vi "S2C_PCIe7841_Proc_AnalogWrite.vi"(8 "Error In":errorcluster, 11 "Data":string) -> (0 "Error Out":errorcluster)   [LabVIEW 2015]
uses:
  S2C_PCIe7841_Proc_Globals.vi
  <vilib>/Utility/error.llb/Error Cluster From Error Code.vi
  <vilib>/rvi/errors/niLvFpgaAdjustHostInterfaceError.vi
  <vilib>/rvi/interface/nirviReadWriteControl/nirviReadWriteControl.xnode
  <vilib>/rvi/interface/Simulation/niFpgaSimulationCallBeginRW.vi
  NiFpgaLv.dll
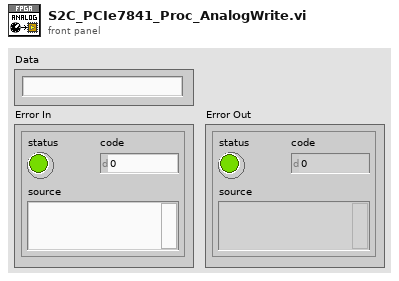
[diagram p1: front panel]
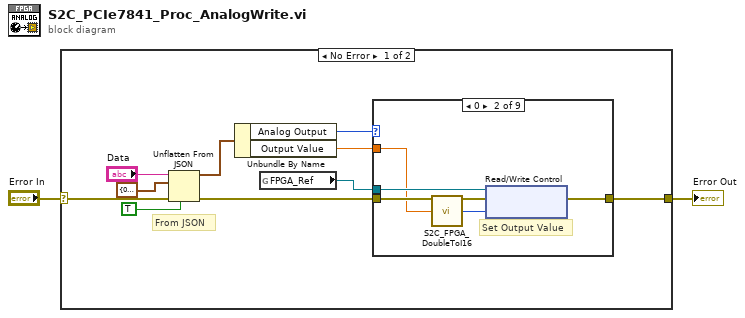
[diagram p0: block diagram]
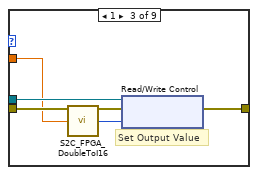
[diagram p3: hidden frame]
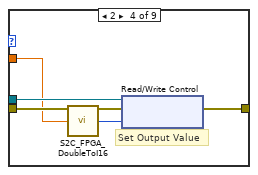
[diagram p4: hidden frame]
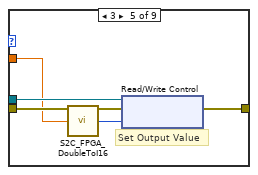
[diagram p5: hidden frame]
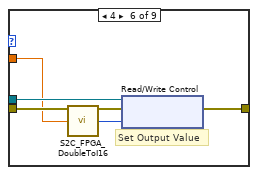
[diagram p6: hidden frame]
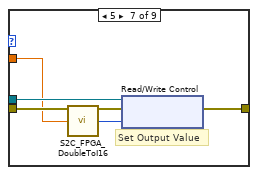
[diagram p7: hidden frame]
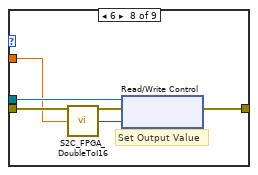
[diagram p8: hidden frame]
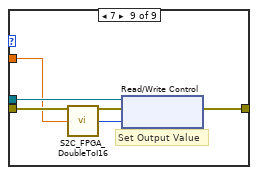
[diagram p9: hidden frame]
diagram:
  n1 = case shown="No Error" "Error In" {
    selector: "Error In" -> [w12 w54]
    tunnel: [w3 w54] -> w1
    frame No Error {
      # "From JSON"
      n2 = Unflatten From JSON(JSON string="Data", type and defaults=cluster{"Analog Output":u16, "Output Value":dbl} {"Analog Output"=0, "Output Value"=0.0}, default null elements? (F)=TRUE, error in (no error)=w12) -> (value=w9:cluster{"Analog Output":u16, "Output Value":dbl}, error out=w7:errorcluster)  [unwired: 3 in]
      n3 = Unbundle By Name(w9) -> ("Analog Output"=w8:u16, "Output Value"=w6:dbl)
      n4 = global read "S2C_PCIe7841_Proc_Globals.vi" "FPGA_Ref"() -> (w5:refnum<k20>)
      n5 = case shown="0" w8 {
        tunnel: w7 -> [w13 w18 w23 w28 w33 w38 w43 w48 w53]
        tunnel: w6 -> [_ w15 w20 w25 w30 w35 w40 w45 w50]
        tunnel: w5 -> [_ w17 w22 w27 w32 w37 w42 w47 w52]
        tunnel: [w13 w16 w21 w26 w31 w36 w41 w46 w51] -> w3
        frame 8, Default {
        }
        frame 0 {
          # "Set Output Value"
          n6 = call "S2C_FPGA_DoubleToI16.vi"("Double In"=w15) -> ("I16 Out"=w14:i16)  [unwired: 4 in]
          n7 = xnode "Read/Write Control"("FPGA VI Reference In"=w17, "error in"=w18, "Conn0/AO0"=w14) -> ("error out"=w16:errorcluster)  [unwired: 1 out]
        }
        frame 1 {
          # "Set Output Value"
          n8 = call "S2C_FPGA_DoubleToI16.vi"("Double In"=w20) -> ("I16 Out"=w19:i16)  [unwired: 4 in]
          n9 = xnode "Read/Write Control"("FPGA VI Reference In"=w22, "error in"=w23, "Conn0/AO1"=w19) -> ("error out"=w21:errorcluster)  [unwired: 1 out]
        }
        frame 2 {
          # "Set Output Value"
          n10 = call "S2C_FPGA_DoubleToI16.vi"("Double In"=w25) -> ("I16 Out"=w24:i16)  [unwired: 4 in]
          n11 = xnode "Read/Write Control"("FPGA VI Reference In"=w27, "error in"=w28, "Conn0/AO2"=w24) -> ("error out"=w26:errorcluster)  [unwired: 1 out]
        }
        frame 3 {
          # "Set Output Value"
          n12 = call "S2C_FPGA_DoubleToI16.vi"("Double In"=w30) -> ("I16 Out"=w29:i16)  [unwired: 4 in]
          n13 = xnode "Read/Write Control"("FPGA VI Reference In"=w32, "error in"=w33, "Conn0/AO3"=w29) -> ("error out"=w31:errorcluster)  [unwired: 1 out]
        }
        frame 4 {
          # "Set Output Value"
          n14 = call "S2C_FPGA_DoubleToI16.vi"("Double In"=w35) -> ("I16 Out"=w34:i16)  [unwired: 4 in]
          n15 = xnode "Read/Write Control"("FPGA VI Reference In"=w37, "error in"=w38, "Conn0/AO4"=w34) -> ("error out"=w36:errorcluster)  [unwired: 1 out]
        }
        frame 5 {
          # "Set Output Value"
          n16 = call "S2C_FPGA_DoubleToI16.vi"("Double In"=w40) -> ("I16 Out"=w39:i16)  [unwired: 4 in]
          n17 = xnode "Read/Write Control"("FPGA VI Reference In"=w42, "error in"=w43, "Conn0/AO5"=w39) -> ("error out"=w41:errorcluster)  [unwired: 1 out]
        }
        frame 6 {
          # "Set Output Value"
          n18 = call "S2C_FPGA_DoubleToI16.vi"("Double In"=w45) -> ("I16 Out"=w44:i16)  [unwired: 4 in]
          n19 = xnode "Read/Write Control"("FPGA VI Reference In"=w47, "error in"=w48, "Conn0/AO6"=w44) -> ("error out"=w46:errorcluster)  [unwired: 1 out]
        }
        frame 7 {
          # "Set Output Value"
          n20 = call "S2C_FPGA_DoubleToI16.vi"("Double In"=w50) -> ("I16 Out"=w49:i16)  [unwired: 4 in]
          n21 = xnode "Read/Write Control"("FPGA VI Reference In"=w52, "error in"=w53, "Conn0/AO7"=w49) -> ("error out"=w51:errorcluster)  [unwired: 1 out]
        }
      }
    }
    frame Error {
    }
  }
  "Error Out" <- w1
